vi "Transfer.Required Buffer Size.vi"(8 "error in (no error)":errorcluster, 11 "Transfer in":refnum<class "Transfer.lvclass">) -> (0 "error out":errorcluster, 2 "required buffer size":u64 format="%d bytes", 3 "Transfer out":refnum<class "Transfer.lvclass">)   [LabVIEW 2017, in "DSF Core.lvlib" / "Transfer.lvclass"]
uses:
  Transfer.lvclass
  Transfer.lvclass/Transfer.ctl
  Shared/VIs/DSF.Data Type.Sizeof.vi
  DSF Core.lvlib
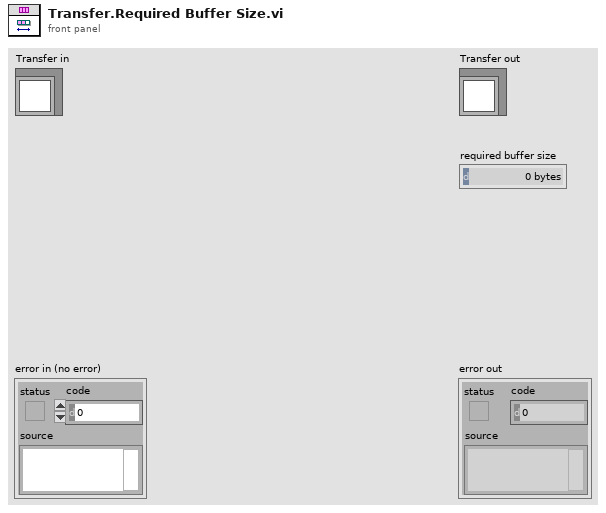
[diagram p1: front panel]
types:
  T1 = typedef "DSF Core.lvlib/DSF Runtime Channel Block.ctl" = cluster{"data type":T2, "count":u64, "buffer offset":u64}
  T2 = typedef "DSF Core.lvlib/Configuration.lvclass/DSF Data Type.ctl" = enum8{"Bool", "SGL", "DBL", "I8", "I16", "I32", "I64", "U8", "U16", "U32", "U64"}
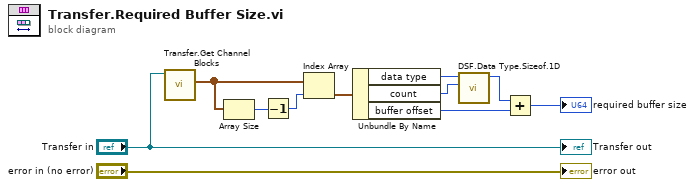
[diagram p0: block diagram]
diagram:
  n1 = call "Transfer.Get Channel Blocks.vi"("Transfer in"="Transfer in") -> ("channel blocks"=w1:T1[])  [unwired: 9 in, 1 out]
  n2 = Array Size(array=w1) -> (size(s)=w9:i32)
  n3 = Decrement(x=w9) -> (x-1=w8:i32)
  n4 = Index Array(array=w1, index=w8) -> (element=w7:T1)
  n5 = Unbundle By Name(w7) -> ("data type"=w6:T2, "count"=w5:u64, "buffer offset"=w3:u64)
  n6 = call "DSF.Data Type.Sizeof.1D.vi"("count"=w5, "data type"=w6) -> ("size in bytes"=w4:u64)  [unwired: 9 in]
  n7 = Add(x=w4, y=w3) -> (x+y=→"required buffer size":u64)
  "error out" <- "error in (no error)"
  "Transfer out" <- "Transfer in"
